vi "用户登录.vi"(8 "error in (no error)":errorcluster caption="错误输入（无错误）", 9 "Password":string caption="密   码:", 11 "UserName":string caption="用户名:") -> (0 "error out":errorcluster caption="错误输出", 1 "ErrorMessage":string, 2 "登录成功":bool)   [LabVIEW 2020]
uses:
  Global.vi
  <vilib>/addons/_JKI.lib/Serialization/JSON/JKI JSON Serialization.lvlib
panel:
  in  "Headers 2":string[][](array[string])=[["Content-Type", "application/json"], ["Connection", "Keep-Alive"], ["User-Agent", "Apache-HttpClient/4.1.1 (java 1.5)"]]
  in  "Headers":string[][](array[string])=[["Content-Type", "application/json"]]
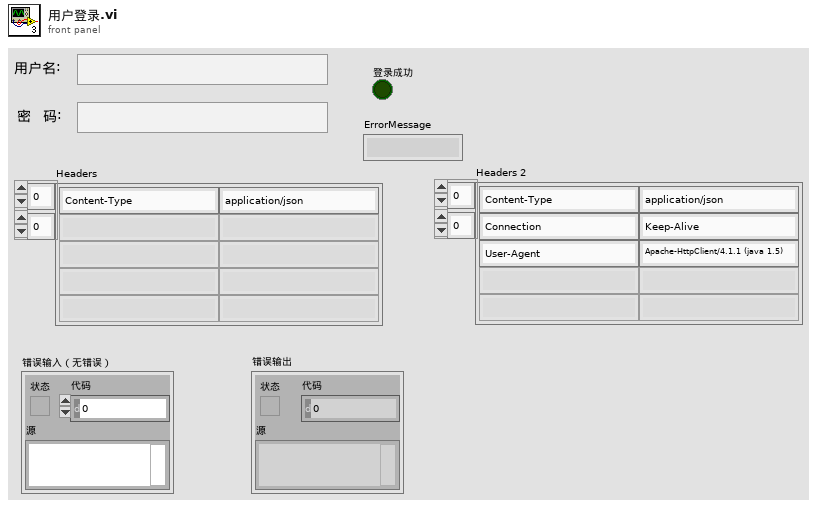
[diagram p1: front panel]
types:
  T1 = cluster{"userName":string, "password":string, "equipmentCode":string}
  T2 = cluster{"接口地址(URL)":string, "用户登录":string, "产品进站":string, "参数采集":string, "产品出站":string, "设备状态":string, "设备编号(equipNum)":string, "站点名称(siteCode)":string, "生产类型(productType)":string, "追溯编号(traceCode)":string}
  T3 = cluster{"data":string, "resCode":i32, "resMsg":string}
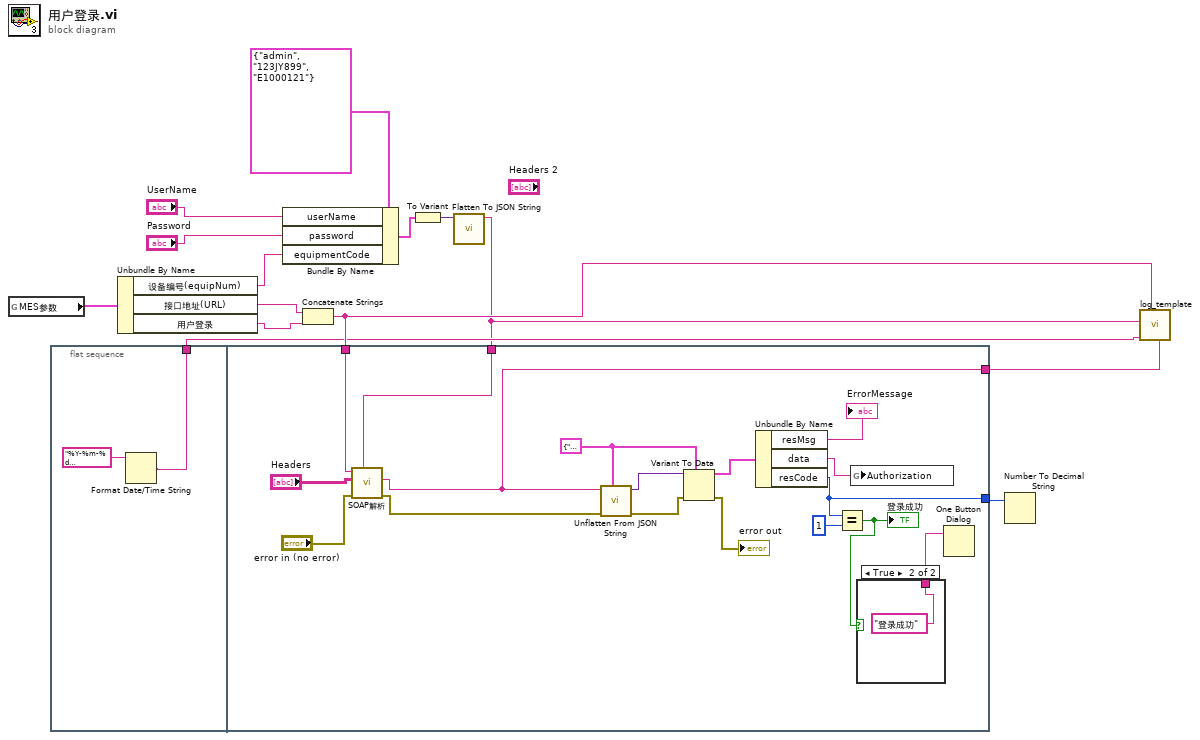
[diagram p0: block diagram]
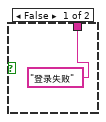
[diagram p2: hidden frame]
diagram:
  n1 = global read "Global.vi" "MES参数"() -> (w14:T2)
  n2 = flat-sequence {
    tunnel: [w15] -> w11
    tunnel: w12 -> [w33]
    tunnel: w4 -> [w29]
    tunnel: [w28] -> w3
    tunnel: [w19] -> w2
    frame #0 {
      n3 = Format Date/Time String(time format string (%c)="%Y-%m-%d %H:%M:%S%3u-->" ("EndTime")) -> (date/time string=w15:string)  [unwired: 2 in]
    }
    frame #1 {
      w25 = T3 {"data"="", "resCode"=0, "resMsg"=""} ("用户登录ctl")
      n4 = call "SOAP解析.vi"("DATA"=w29, "错误输入（无错误）"="error in (no error)", "Headers"="Headers", "URL"=w33) -> ("错误输出"=w26:errorcluster, "body"=w19:string)  [unwired: 5 in, 1 out]
      n5 = call <vilib>:"Unflatten From JSON String.vi"("Type and Defaults"=w25, "error in (no error)"=w26, "JSON String"=w19) -> ("error out"=w24:errorcluster, "Variant"=w27:variant)  [unwired: 7 in]
      n6 = Variant To Data(error in=w24, type=w25, Variant=w27) -> (data=w32:T3, error out=→"error out":errorcluster)
      n7 = Unbundle By Name(w32) -> ("resMsg"=→"ErrorMessage":string, "data"=w20:string, "resCode"=w28:i32)
      n8 = Equal?(x=w28, y=1) -> (x = y?=w18:bool)
      "登录成功" <- w18
      n9 = global write "Global.vi" "Authorization"(w20) -> ()
      n10 = case shown="True" w18 {
        tunnel: ["登录失败" "登录成功"] -> w17
        frame False {
        }
        frame True {
        }
      }
      n11 = One Button Dialog(message=w17) -> ()  [unwired: 1 in, 1 out]
    }
  }
  n12 = Unbundle By Name(w14) -> ("设备编号(equipNum)"=w7:string, "接口地址(URL)"=w1:string, "用户登录"=w13:string)
  n13 = Bundle By Name(cluster=T1 {"userName"="admin", "password"="123JY899", "equipmentCode"="E1000121"} ("用户登录ctl"), "userName"="UserName", "password"="Password", "equipmentCode"=w7) -> (w6:T1)
  n14 = Concatenate Strings(w1, w13) -> (w12:string)
  n15 = To Variant(anything=w6) -> (Variant=w5:variant)
  n16 = call <vilib>:"Flatten To JSON String.vi"("Variant"=w5) -> ("JSON String"=w4:string)  [unwired: 9 in, 1 out]
  n17 = Number To Decimal String(number=w3) -> ()  [unwired: 1 in, 1 out]
  n18 = call "log_template.vi"("接收报文"=w2, "URL"=w12, "StartTime"=w11, "发送报文"=w4) -> ()  [unwired: 8 in]
